vi "TalkTracker.vi"(0 "PORT NAME":string="Inlet_Heaters", 1 "Set":enum16{"Set", "Read"}(ring), 2 "Channel Name":string, 3 "Value to set":dbl, 5 "MODULE ADDRESS":i32=1, 9 "LOCATION":i32=15, 11 "NO. LOCATIONS":i32=1, 12 "Analogue":enum16{"Logic", "Analogue"}(ring), 13 "Timeout/ms":u32=500) -> (4 "Response":string=" ON\r\n", 10 "Good Set?":bool, 15 "Comment out":string)   [LabVIEW 2011]
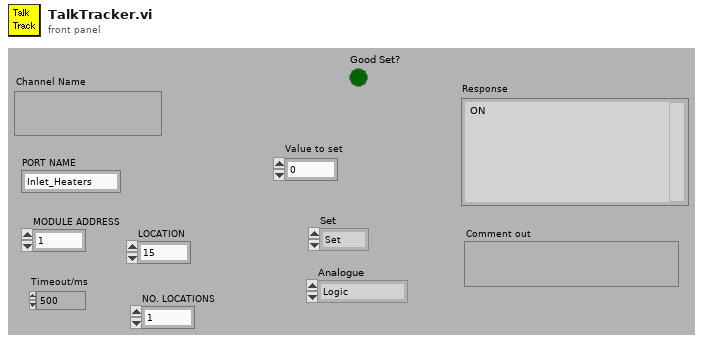
[diagram p1: front panel]
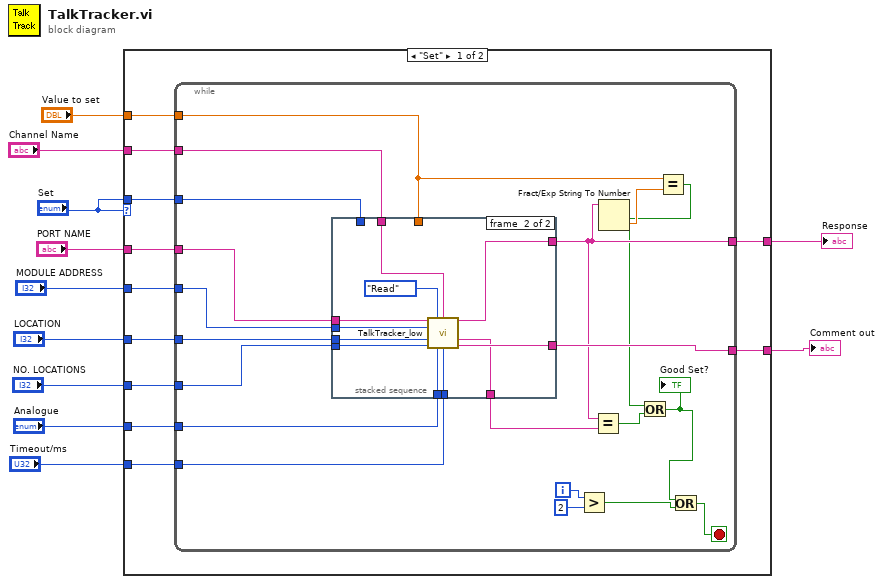
[diagram p0: block diagram]
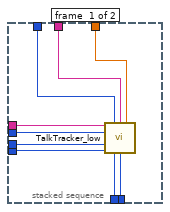
[diagram p2: hidden frame]
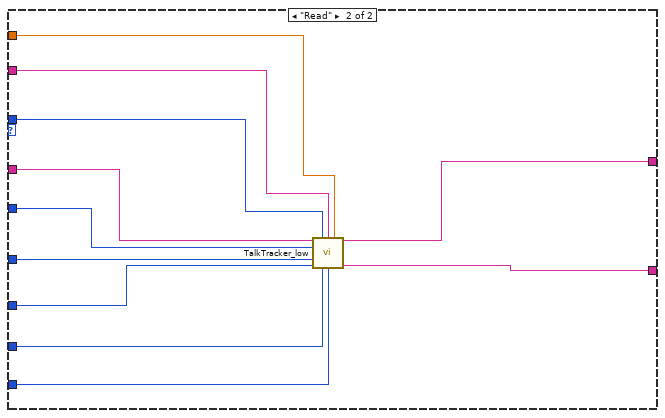
[diagram p3: hidden frame]
diagram:
  n1 = case shown="\"Set\"" "Set" {
    tunnel: "Set" -> [w22 w73]
    tunnel: "Value to set" -> [w21 w72]
    tunnel: "Channel Name" -> [w20 w71]
    tunnel: "PORT NAME" -> [w19 w70]
    tunnel: "MODULE ADDRESS" -> [w18 w69]
    tunnel: "LOCATION" -> [w17 w68]
    tunnel: "NO. LOCATIONS" -> [w16 w67]
    tunnel: "Analogue" -> [w15 w66]
    tunnel: "Timeout/ms" -> [w14 w65]
    tunnel: [w13 w63] -> w2
    tunnel: [w12 w64] -> w1
    frame "Set" {
      n2 = while {
        tunnel: w22 -> [w42]
        tunnel: w21 -> [w30]
        tunnel: w20 -> [w35]
        tunnel: w19 -> [w36]
        tunnel: w18 -> [w37]
        tunnel: w17 -> [w38]
        tunnel: w16 -> [w39]
        tunnel: w15 -> [w40]
        tunnel: w14 -> [w41]
        tunnel: [w34] -> w13
        tunnel: [w32] -> w12
        i -> [w27]
        stop <- w23 stop-if-true
        n3 = stacked-sequence {
          tunnel: w42 -> [w51 _]
          tunnel: w30 -> [w50 _]
          tunnel: w41 -> [w49 w62]
          tunnel: w40 -> [w48 w61]
          tunnel: w39 -> [w47 w60]
          tunnel: w38 -> [w46 w59]
          tunnel: w37 -> [w45 w58]
          tunnel: w36 -> [w44 w57]
          tunnel: w35 -> [w43 w56]
          tunnel: [_ w54] -> w34
          tunnel: [_ w53] -> w32
          tunnel: [_ w52] -> w33
          frame #0 {
            n4 = call "TalkTracker_low.vi"("PORT NAME"=w44, "Set"=w51, "Channel Name"=w43, "Value to set"=w50, "MODULE ADDRESS"=w45, "LOCATION"=w46, "NO. LOCATIONS"=w47, "Analogue"=w48, "Timeout/ms"=w49) -> ()  [unwired: 7 out]
          }
          frame #1 {
            n5 = call "TalkTracker_low.vi"("PORT NAME"=w57, "Set"=enum16{"Set", "Read"}."Read", "Channel Name"=w56, "MODULE ADDRESS"=w58, "LOCATION"=w59, "NO. LOCATIONS"=w60, "Analogue"=w61, "Timeout/ms"=w62) -> ("Response"=w53:string, "Set String"=w52:string, "Comment out"=w54:string)  [unwired: 1 in, 4 out]
          }
        }
        n6 = Greater?(x=w27, y=2) -> (0:w25:bool)
        n7 = Equal?(x=w32, y=w33) -> (x = y?=w29:bool)
        n8 = Fract/Exp String To Number(string=w32) -> (number=w31:dbl)  [unwired: 4 out]
        n9 = Equal?(x=w30, y=w31) -> (x = y?=w28:bool)
        n10 = Or(x=w28, y=w29) -> (x .or. y?=w24:bool)
        "Good Set?" <- w24
        n11 = Or(x=w24, y=w25) -> (x .or. y?=w23:bool)
      }
    }
    frame "Read" {
      n12 = call "TalkTracker_low.vi"("PORT NAME"=w70, "Set"=w73, "Channel Name"=w71, "Value to set"=w72, "MODULE ADDRESS"=w69, "LOCATION"=w68, "NO. LOCATIONS"=w67, "Analogue"=w66, "Timeout/ms"=w65) -> ("Response"=w64:string, "Comment out"=w63:string)  [unwired: 5 out]
    }
  }
  "Response" <- w1
  "Comment out" <- w2
